vi "setWriteFIFO.vi"(10 "WriteFIFO":refnum<class "IWriteFIFO.lvclass">, 11 "RTHealthAndStatus in":refnum<class "RTHealthAndStatus.lvclass">) -> (3 "RTHealthAndStatus out":refnum<class "RTHealthAndStatus.lvclass">)   [LabVIEW 2015, in "RTHealthAndStatus.lvlib" / "RTHealthAndStatus.lvclass"]
uses:
  RTHealthAndStatus.lvclass
  Common_RT_FPGA/IWriteFIFO/IWriteFIFO.lvclass
  RTHealthAndStatus.lvclass/RTHealthAndStatus.ctl
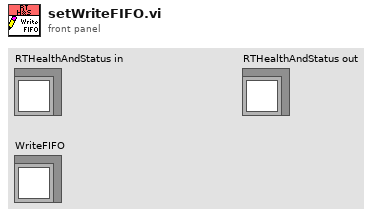
[diagram p1: front panel]
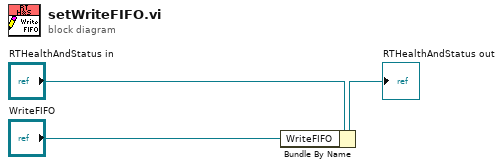
[diagram p0: block diagram]
diagram:
  n1 = Bundle By Name(cluster="RTHealthAndStatus in", "WriteFIFO"="WriteFIFO") -> (→"RTHealthAndStatus out":refnum<class "RTHealthAndStatus.lvclass">)
